vi "总量测量7.24.vi"() -> ()   [LabVIEW 2015]
panel:
  out "Boolean":bool
  out "data out":string
  out "*(type *) &x":u32[](array[numeric])
  out "Waveform Chart":dbl[](graph)
  out "# of Received":i32
  out "# of Sent":i32
  in  "stop":bool
  # "此程序将一直等待客户端的连接，直到客户端请求连接后才发送并读取数据。"
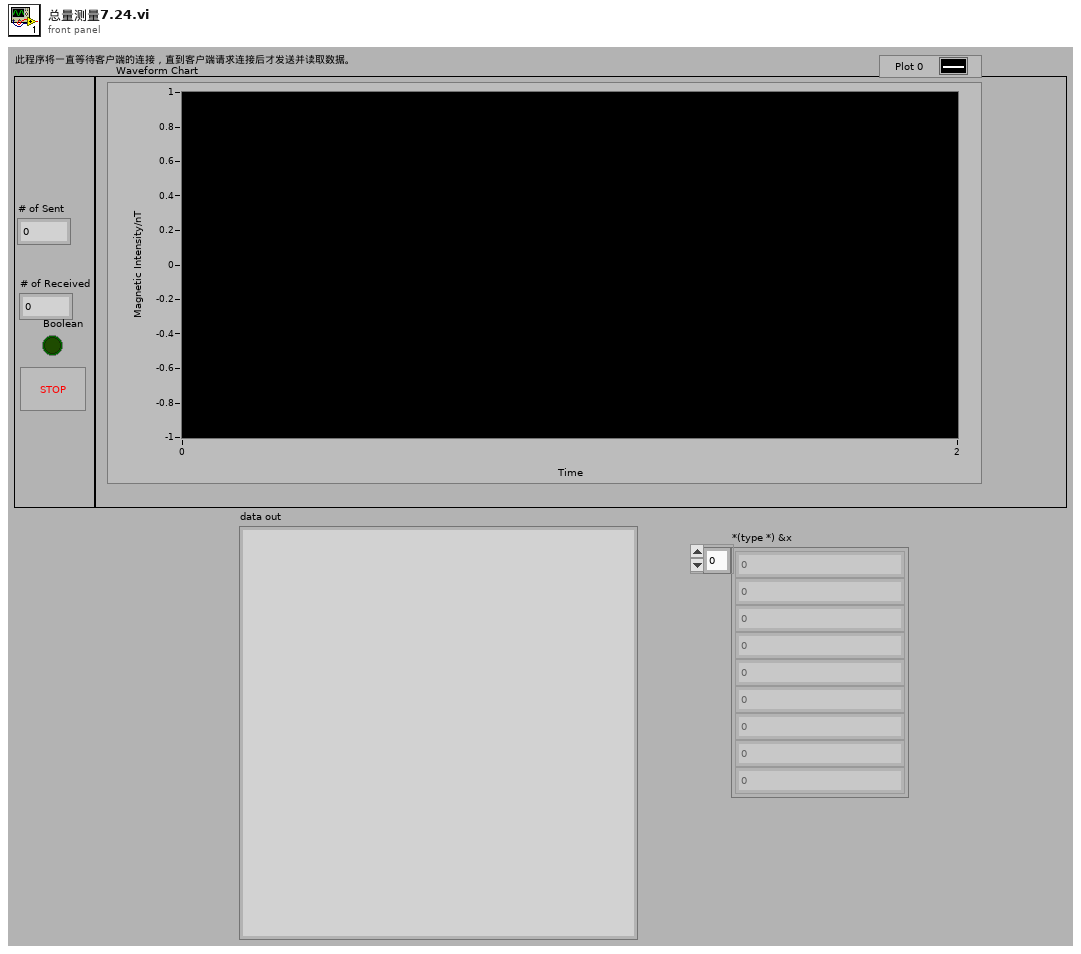
[diagram p1: front panel]
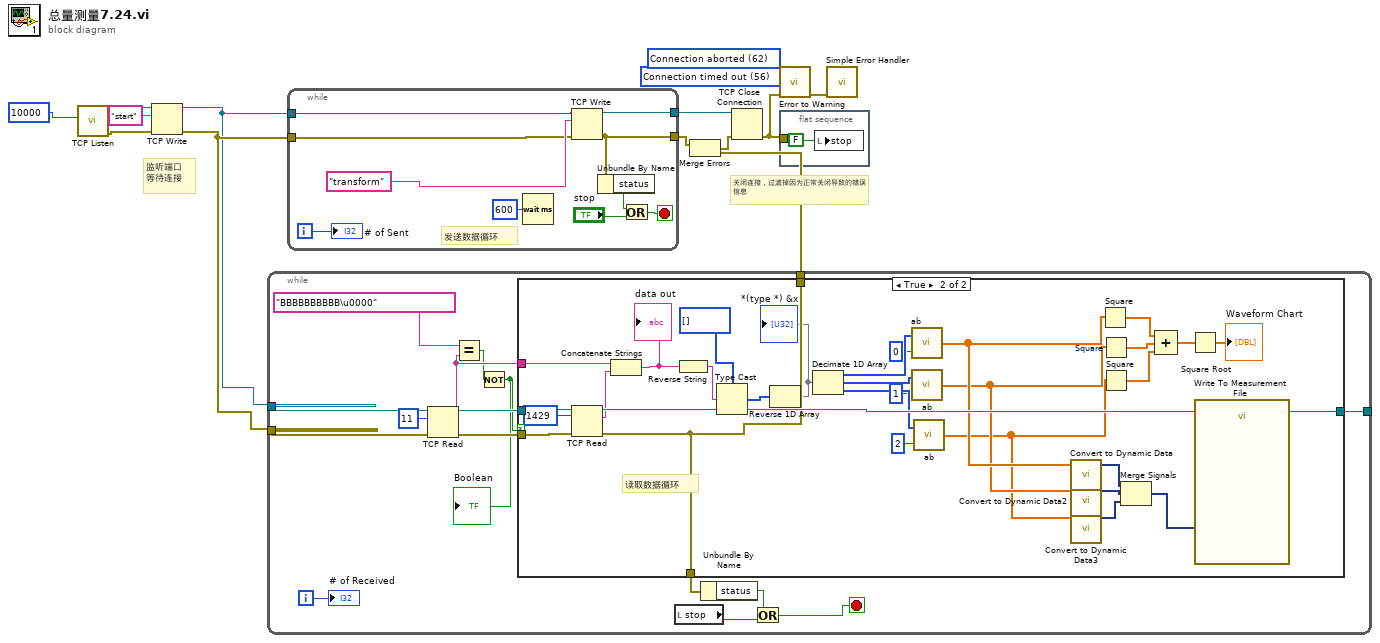
[diagram p0: block diagram]
diagram:
  w11 = 56 items=["No Error", "Argument Error", "Memory Full", "Out of Zone", "End of File", "File Already Open", "Generic File IO Error", "File Not Found", "File Permission Error", "Disk Full", "Duplicate Path", "Too Many Files Open", "Not Enabled", "Resource File Not Found", "Cannot Add Resource", "Resource Not Found", "Image Not Found", "Image Memory Error", "Pen Does Not Exist", "Config Bad Type", "Config Token Not Found", "Config Parse Error", "Config Memory Error", "Bad External Code Format", "Bad External Code Offset", "External Code Not Present", "Null Window", "Destroy Window Mixup", "Null Menu", "Print Aborted", "Bad Print Record", "Print Driver Error", "Windows Error During Print", "Memory Error During Print", "Print Dialog Error", "Generic Print Error", "Invalid Device Refnum", "Device Not Found", "Device Parameter Error", "Device Unit Error", "Can't Open Device", "Device Call Aborted", "Generic Error", "Cancelled By User", "Object ID Too Low", "Object ID Too High", "Object Not In Heap", "Unknown Heap", "Bad DefProc ID", "DefProc Not In Table", "Message Out Of Range", "Null Method", "Unknown Message", "Manager Call Not Supported", "Bad address", "Connection In progress", "Connection timed out", "Connection is already in progress", "Network attribute not supported", "Network error", "Address in use", "System out of memory", "Connection aborted", "Connection refused", "Connection is not connected", "Connection is already connected", "Connection closed", "Initialize error (interapplication manager)", "Bad occurrence", "Wait on unbound occurrence handler", "Occurrence queue overflow", "Bad path", "Semaphore not signaled", "Unrecognized type (interapplication manager)"] ("2nd Error to Convert")
  w12 = 62 items=["No Error", "Argument Error", "Memory Full", "Out of Zone", "End of File", "File Already Open", "Generic File IO Error", "File Not Found", "File Permission Error", "Disk Full", "Duplicate Path", "Too Many Files Open", "Not Enabled", "Resource File Not Found", "Cannot Add Resource", "Resource Not Found", "Image Not Found", "Image Memory Error", "Pen Does Not Exist", "Config Bad Type", "Config Token Not Found", "Config Parse Error", "Config Memory Error", "Bad External Code Format", "Bad External Code Offset", "External Code Not Present", "Null Window", "Destroy Window Mixup", "Null Menu", "Print Aborted", "Bad Print Record", "Print Driver Error", "Windows Error During Print", "Memory Error During Print", "Print Dialog Error", "Generic Print Error", "Invalid Device Refnum", "Device Not Found", "Device Parameter Error", "Device Unit Error", "Can't Open Device", "Device Call Aborted", "Generic Error", "Cancelled By User", "Object ID Too Low", "Object ID Too High", "Object Not In Heap", "Unknown Heap", "Bad DefProc ID", "DefProc Not In Table", "Message Out Of Range", "Null Method", "Unknown Message", "Manager Call Not Supported", "Bad address", "Connection In progress", "Connection timed out", "Connection is already in progress", "Network attribute not supported", "Network error", "Address in use", "System out of memory", "Connection aborted", "Connection refused", "Connection is not connected", "Connection is already connected", "Connection closed", "Initialize error (interapplication manager)", "Bad occurrence", "Wait on unbound occurrence handler", "Occurrence queue overflow", "Bad path", "Semaphore not signaled", "Unrecognized type (interapplication manager)"] ("1st Error to Convert")
  # "关闭连接，过滤掉因为正常关闭导致的错误信息"
  # "监听端口\n等待连接"
  n1 = call <vilib>:"TCP Listen.vi"("port"=10000) -> ("error out"=w6:errorcluster, "connection ID"=w7:refnum<k5>)  [unwired: 6 in, 3 out]
  n2 = TCP Write(connection ID=w7, data in="start", error in (no error)=w6) -> (connection ID out=w1:refnum<k5>, error out=w2:errorcluster)  [unwired: 1 in, 1 out]
  n3 = while {
    tunnel: w1 -> [w27]
    tunnel: w2 -> [w24]
    tunnel: [w30] -> _
    tunnel: [w28] -> w3
    i -> [w29]
    stop <- w17 stop-if-true
    n4 = TCP Read(connection ID=w27, bytes to read=11, error in (no error)=w24) -> (connection ID out=w26:refnum<k5>, data out=w22:string, error out=w25:errorcluster)  [unwired: 2 in]
    n5 = Equal?(x="BBBBBBBBBB\u0000", y=w22) -> (x = y?=w20:bool)
    n6 = Not(x=w20) -> (.not. x?=w15:bool)
    "Boolean" <- w15
    n7 = case shown="True" w15 {
      tunnel: [w32 w62] -> w30
      tunnel: [w31 w48] -> w28
      tunnel: w26 -> [w32 w52]
      tunnel: w25 -> [w31 w51]
      tunnel: w22 -> [_ w47]
      tunnel: [w31 w48] -> w16
      frame False {
      }
      frame True {
        # "读取数据循环"
        n8 = TCP Read(connection ID=w52, bytes to read=1429, error in (no error)=w51) -> (connection ID out=w62:refnum<k5>, data out=w49:string, error out=w48:errorcluster)  [unwired: 2 in]
        n9 = Concatenate Strings(w47, w49) -> (w50:string)
        "data out" <- w50
        n10 = Reverse String(1:w50) -> (0:w59:string)
        n11 = Type Cast(type=u32[] [], x=w59) -> (*(type *) &x=w46:u32[])
        n12 = Reverse 1D Array(array=w46) -> (reversed array=w45:u32[])
        "*(type *) &x" <- w45
        n13 = Decimate 1D Array(w45) -> (w41:u32[], w40:u32[], w39:u32[])
        n14 = call "ab.vi"("Numeric 2"=0, "Array"=w41) -> ("Array 2"=w35:dbl[])
        n15 = call "ab.vi"("Numeric 2"=1, "Array"=w40) -> ("Array 2"=w34:dbl[])
        n16 = call "ab.vi"("Numeric 2"=2, "Array"=w39) -> ("Array 2"=w33:dbl[])
        n17 = call "Convert to Dynamic Data"("Array"=w35) -> ("Dynamic Data Type"=w53:dynamicdata)  [unwired: 3 in]
        n18 = call "Convert to Dynamic Data2"("Array"=w34) -> ("Dynamic Data Type"=w43:dynamicdata)  [unwired: 3 in]
        n19 = call "Convert to Dynamic Data3"("Array"=w33) -> ("Dynamic Data Type"=w42:dynamicdata)  [unwired: 3 in]
        n20 = Square(x=w35) -> (x^2=w58:dbl[])
        n21 = Square(x=w34) -> (x^2=w57:dbl[])
        n22 = Square(x=w33) -> (x^2=w56:dbl[])
        n23 = Merge Signals(w53, w43, w42) -> (w54:dynamicdata)
        n24 = Compound Arithmetic op=ADD(w58, w57, w56) -> (w55:dbl[])
        n25 = Square Root(x=w55) -> (sqrt(x)=→"Waveform Chart":dbl[])
        n26 = call "Write To Measurement File"("Signals"=w54) -> ()  [unwired: 16 in, 3 out]
      }
    }
    n27 = local read "stop"() -> (w19:bool)
    n28 = Unbundle By Name(w16) -> ("status"=w18:bool)
    n29 = Or(x=w18, y=w19) -> (x .or. y?=w17:bool)
    "# of Received" <- w29
  }
  n30 = while {
    tunnel: w2 -> [w64]
    tunnel: w1 -> [w63]
    tunnel: [w69] -> w10
    tunnel: [w68] -> w14
    i -> [w66]
    stop <- w70 stop-if-true
    # "发送数据循环"
    n31 = Wait (ms)(milliseconds to wait=u32 600) -> ()  [unwired: 1 out]
    n32 = TCP Write(connection ID=w63, data in="transform", error in (no error)=w64) -> (connection ID out=w68:refnum<k5>, error out=w69:errorcluster)  [unwired: 1 in, 1 out]
    n33 = Unbundle By Name(w69) -> ("status"=w71:bool)
    n34 = Or(x=w71, y="stop") -> (x .or. y?=w70:bool)
    "# of Sent" <- w66
  }
  n35 = Merge Errors(w10, w3) -> (w9:errorcluster)
  n36 = TCP Close Connection(connection ID=w14, error in (no error)=w9) -> (error out=w8:errorcluster)  [unwired: 1 in, 1 out]
  n37 = call <vilib>:"Error to Warning.vi"("1st Error to Convert"=w12, "2nd Error to Convert"=w11, "error in"=w8) -> ("warning out"=w13:errorcluster)  [unwired: 12 in]
  n38 = flat-sequence {
    tunnel: w8 -> [_]
    frame #0 {
      n39 = local write "stop"(FALSE ("stop")) -> ()
    }
  }
  n40 = call <vilib>:"Simple Error Handler.vi"("error in (no error)"=w13) -> ()  [unwired: 4 in, 5 out]
